vi "AixplorerMultiplexLoad.vi"() -> ()   [LabVIEW 2015]
uses:
  Tek shared libraries/ArbitraryFunctions/VImode.vi
  General Libraries/Sequences.lvlib
  Tek shared libraries/ArbitraryFunctions.lvlib
panel:
  in  "Stop Button":bool
  out "error out":errorcluster
  in  "resource name":refnum<k15>
  in  "?":enum32{"define waveforms", "load sequence"}(tab)
  in  "clear waveforms":bool
  out "Waveform Graph":dbl[][](graph)
  in  "define waveform":bool
  in  "Sequence Loop Initialization":T1(array[cluster])=[{"min"=0.0, "step"=0.25, "max"=1.0, "name"="Phase"}, {"min"=1.0, "step"=1.0, "max"=3.0, "name"="Harmonic"}]
  in  "Frequency LOW fundamental (Hz)":dbl=32467.5
  out "list waveform":string[][](table) caption="Loop variable"
  in  "N point":i32=960
  out "samplr rate":dbl
  in  "load sequence":bool
  in  "update voltage":bool
  in  "High Voltage (0.25)":dbl=0.5 format="%#_13g"
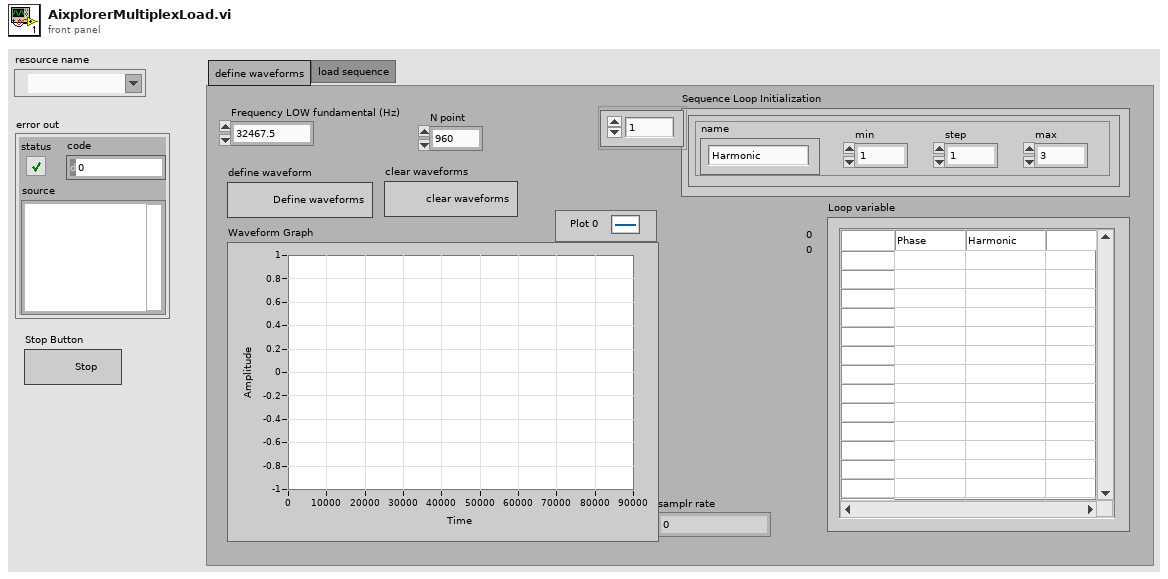
[diagram p1: front panel]
types:
  T1 = cluster{"min":dbl, "step":dbl, "max":dbl, "name":string}[]
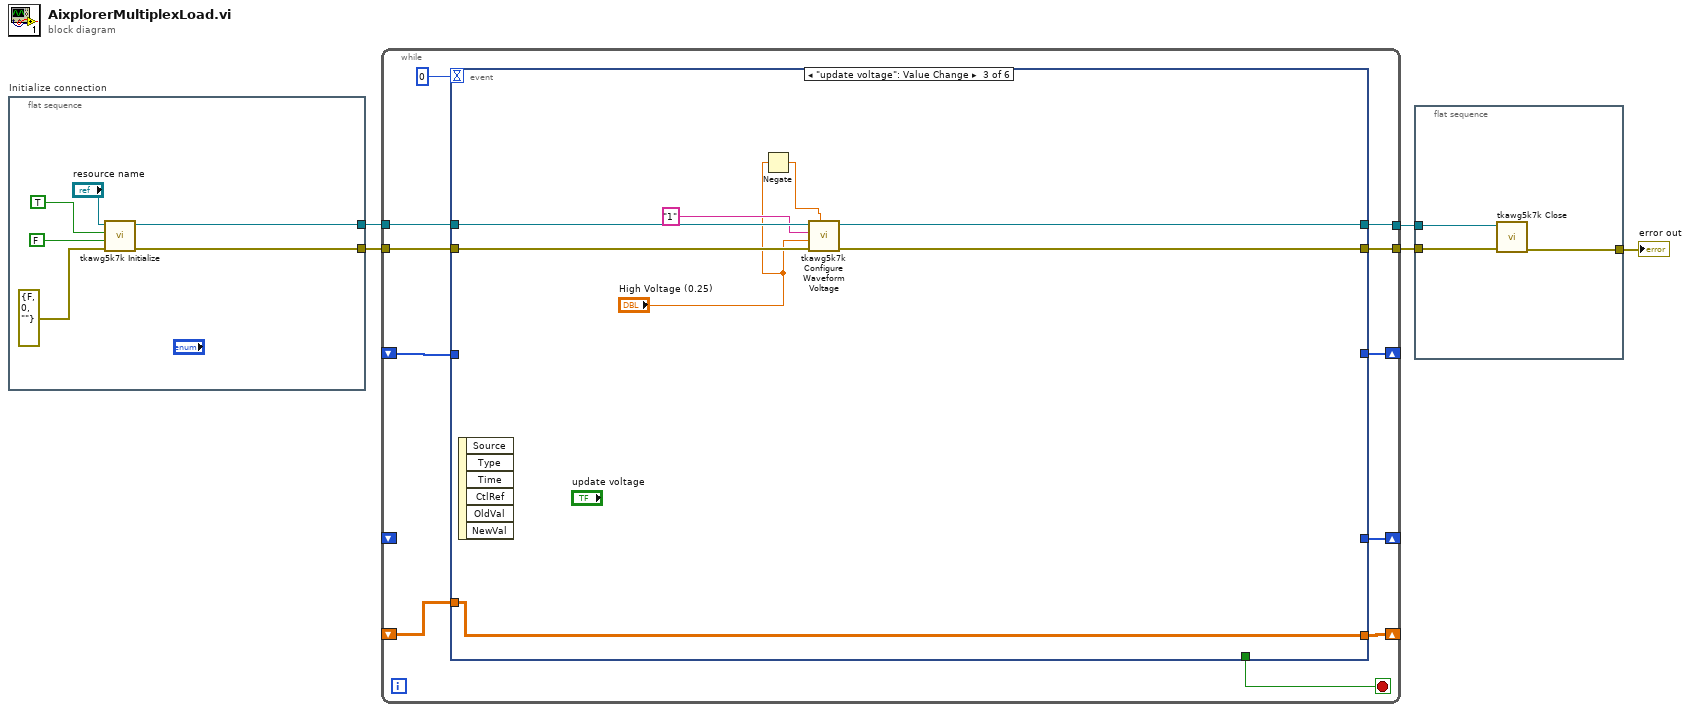
[diagram p0: block diagram]
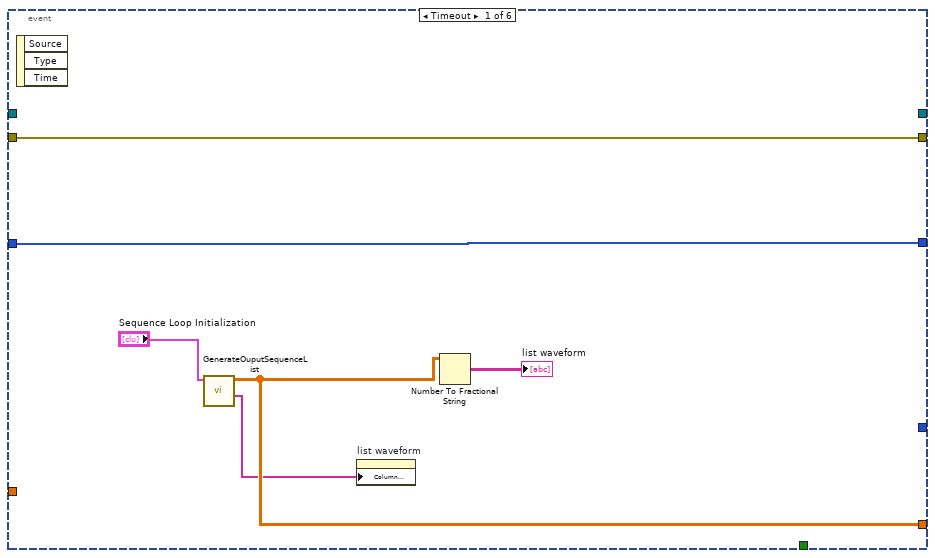
[diagram p2: hidden frame]
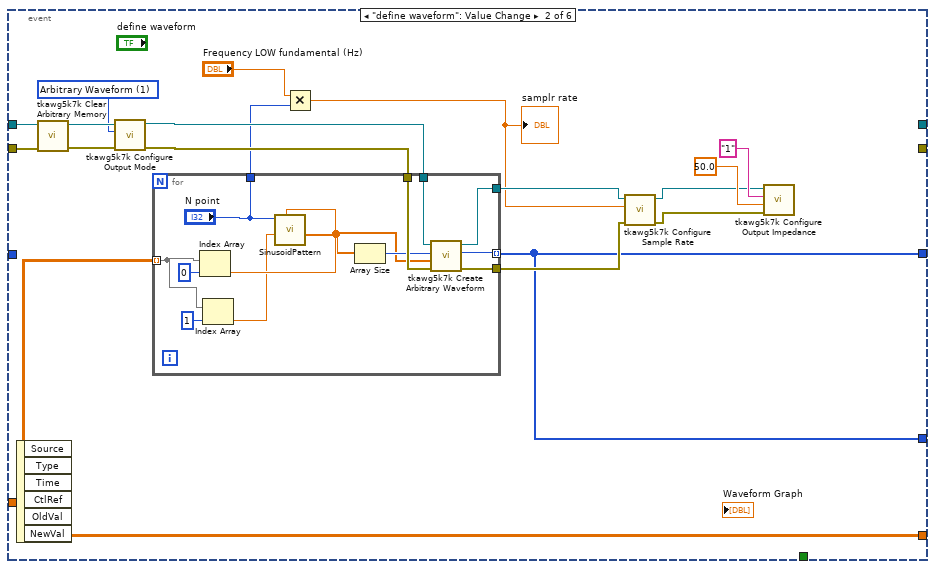
[diagram p3: hidden frame]
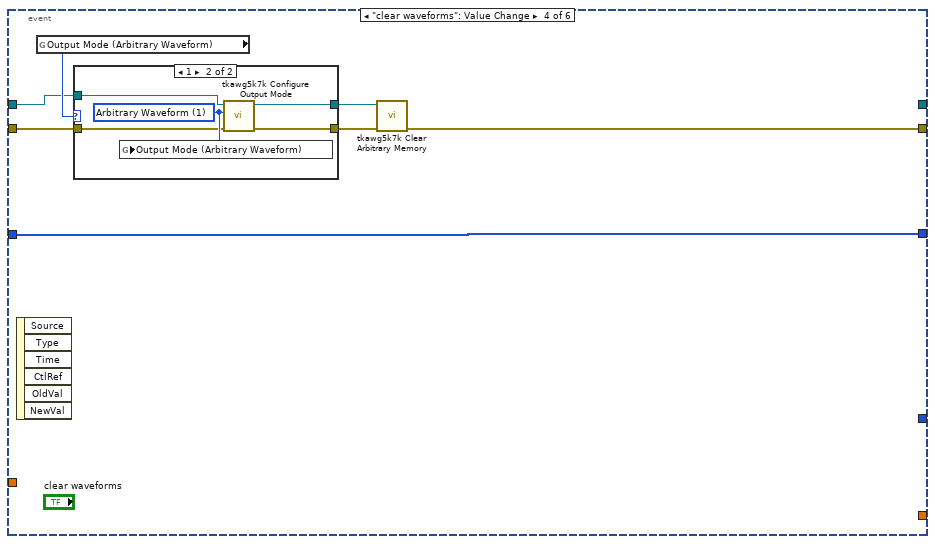
[diagram p4: hidden frame]
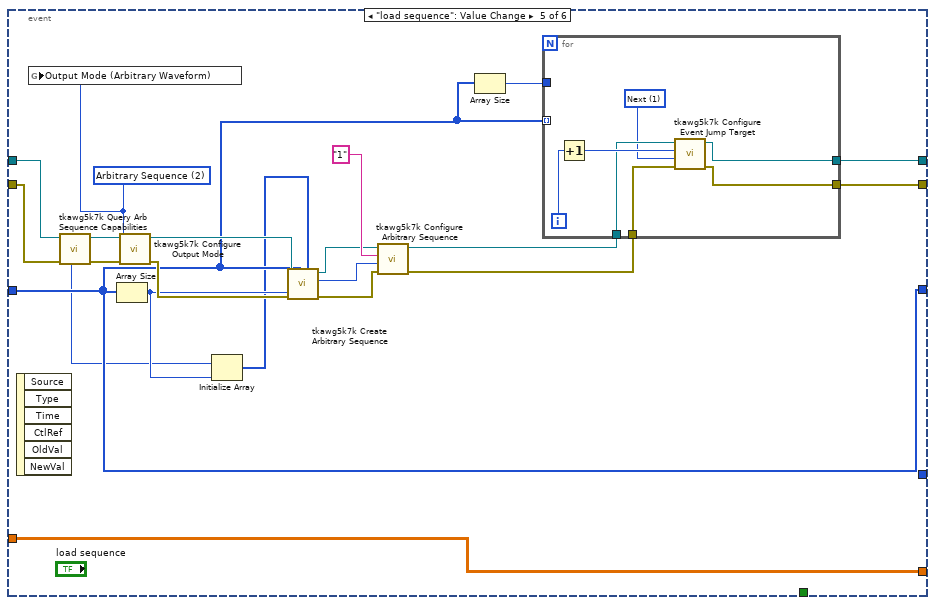
[diagram p6: hidden frame]
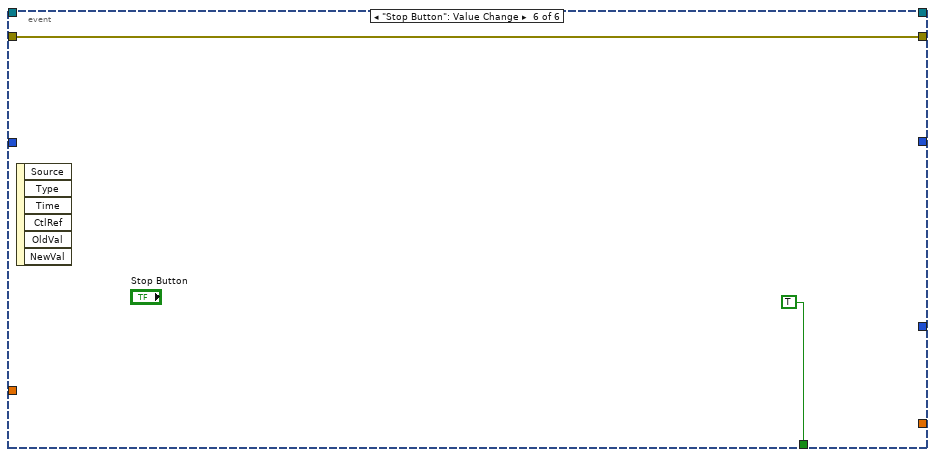
[diagram p7: hidden frame]
diagram:
  n1 = flat-sequence "Initialize connection" {
    tunnel: [w7] -> w5
    tunnel: [w6] -> w4
    frame #0 {
      n2 = call <instrlib>:"tkawg5k7k Initialize.vi"("error in (no error)"=errorcluster {"status"=FALSE, "code"=0, "source"=""}, "Reset Device (Yes)"=FALSE, "ID Query (Yes)"=TRUE, "resource name"="resource name") -> ("error out"=w6:errorcluster, "instrument handle out"=w7:refnum<k15>)  [unwired: 6 in]
    }
  }
  n3 = while {
    tunnel: w5 -> [w21]
    tunnel: w4 -> [w20]
    tunnel: [w22] -> w3
    tunnel: [w19] -> w2
    shift-right: [w16] -> _
    shift-left: _ -> [w15]
    shift-right: [w14] -> _
    shift-left: _ -> [w13]
    shift-right: [w12] -> _
    shift-left: _ -> [_]
    stop <- w17 stop-if-true
    n4 = event shown="[2] \"update voltage\": Value Change" {
      selector: _ -> [_ _ _ _ _ _]
      dyn-events: _ -> [_ _ _ _ _ _]
      timeout: 0 -> [_ _ _ _ _ _]
      tunnel: [_ _ w63 _ w91 _] -> w22
      tunnel: w21 -> [_ w45 w66 w73 w88 _]
      tunnel: w20 -> [w28 w44 w65 w72 w87 w110]
      tunnel: [w28 _ w62 w69 w94 w110] -> w19
      tunnel: [_ _ _ _ _ TRUE] -> w17
      tunnel: [w25 w46 w67 _ w102 _] -> w16
      tunnel: w15 -> [_ w46 w67 _ w102 _]
      tunnel: [w26 w32 _ w71 w93 _] -> w14
      tunnel: w13 -> [w26 _ _ w71 w93 _]
      tunnel: [_ w32 _ _ _ _] -> w12
      event Timeout {
        n5 = event-data() -> ()  [unwired: 1 in, 3 out]
        n6 = call "GenerateOuputSequenceList.vi"("input parameters"="Sequence Loop Initialization") -> ("output Names"=w23:string[], "output array"=w25:dbl[][])  [unwired: 9 in]
        n7 = property on="list waveform" class="Tbl (strict)"("Column Headers[]"=w23) -> ()  [unwired: 2 in, 2 out]
        n8 = Number To Fractional String(number=w25) -> (F-format string=→"list waveform":string[][])  [unwired: 3 in]
      }
      event "define waveform": Value Change {
        w39 = 1 items=["Arbitrary Waveform"=1, "Arbitrary Sequence"=2] ("Output Mode (Arbitrary Waveform)")
        n9 = event-data() -> ()  [unwired: 1 in, 6 out]
        n10 = call <instrlib>:"tkawg5k7k Clear Arbitrary Memory.vi"("error in (no error)"=w44, "instrument handle"=w45) -> ("error out"=w43:errorcluster, "instrument handle out"=w41:refnum<k15>)  [unwired: 8 in]
        n11 = call <instrlib>:"tkawg5k7k Configure Output Mode.vi"("error in (no error)"=w43, "Output Mode (Arbitrary Waveform)"=w39, "instrument handle"=w41) -> ("error out"=w42:errorcluster, "instrument handle out"=w40:refnum<k15>)  [unwired: 7 in]
        n12 = for {
          tunnel: w46 -> [w57] mode=indexing
          tunnel: w40 -> [w56]
          tunnel: w42 -> [w55]
          tunnel: [w53] -> w35
          tunnel: [w52] -> w36
          tunnel: [w51] -> w32 mode=indexing
          tunnel: ["N point"] -> w30
          n13 = Index Array(array=w57, index=0) -> (element=w50:dbl)
          n14 = Index Array(array=w57, index=1) -> (element=w49:dbl)
          n15 = call "SinusoidPattern.vi"("Phase (2pi unit)"=w50, "Nrep"=w49, "N point"="N point") -> ("Unit Pattern"=w48:dbl[])  [unwired: 7 in, 1 out]
          n16 = Array Size(array=w48) -> (size(s)=w54:i32)
          n17 = call <instrlib>:"tkawg5k7k Create Arbitrary Waveform.vi"("error in (no error)"=w55, "Waveform Data Array"=w48, "Waveform Size"=w54, "instrument handle"=w56) -> ("error out"=w53:errorcluster, "Waveform Handle"=w51:i32, "instrument handle out"=w52:refnum<k15>)  [unwired: 5 in]
        }
        n18 = Multiply(x="Frequency LOW fundamental (Hz)", y=w30) -> (x*y=w29:dbl)
        "samplr rate" <- w29
        n19 = call <instrlib>:"tkawg5k7k Configure Sample Rate.vi"("error in (no error)"=w35, "Sample Rate (5.0e+8)"=w29, "instrument handle"=w36) -> ("error out"=w34:errorcluster, "instrument handle out"=w33:refnum<k15>)  [unwired: 7 in]
        n20 = call <instrlib>:"tkawg5k7k Configure Output Impedance.vi"("error in (no error)"=w34, "Impedance (50.0)"=50.0, "Channel Name (\"1\")"="1" ("Channel Name (\"1\")"), "instrument handle"=w33) -> ()  [unwired: 6 in, 2 out]
      }
      event "update voltage": Value Change {
        n21 = event-data() -> ()  [unwired: 1 in, 6 out]
        n22 = Negate(x="High Voltage (0.25)") -> (-x=w60:dbl)
        n23 = call <instrlib>:"tkawg5k7k Configure Waveform Voltage.vi"("Low Voltage (-0.25)"=w60, "error in (no error)"=w65, "High Voltage (0.25)"="High Voltage (0.25)", "Channel Name (\"1\")"="1" ("Channel Name (\"1\")"), "instrument handle"=w66) -> ("error out"=w62:errorcluster, "instrument handle out"=w63:refnum<k15>)  [unwired: 5 in]
      }
      event "clear waveforms": Value Change {
        n24 = event-data() -> ()  [unwired: 1 in, 6 out]
        n25 = global read "VImode.vi" "Output Mode (Arbitrary Waveform)"() -> (w74:i32)
        n26 = case shown="1" w74 {
          tunnel: w73 -> [w76 w80]
          tunnel: w72 -> [w75 w79]
          tunnel: [w76 w78] -> w68
          tunnel: [w75 w77] -> w70
          frame 0, Default {
          }
          frame 1 {
            w81 = 1 items=["Arbitrary Waveform"=1, "Arbitrary Sequence"=2] ("Output Mode (Arbitrary Waveform)")
            n27 = global write "VImode.vi" "Output Mode (Arbitrary Waveform)"(w81) -> ()
            n28 = call <instrlib>:"tkawg5k7k Configure Output Mode.vi"("error in (no error)"=w79, "Output Mode (Arbitrary Waveform)"=w81, "instrument handle"=w80) -> ("error out"=w77:errorcluster, "instrument handle out"=w78:refnum<k15>)  [unwired: 7 in]
          }
        }
        n29 = call <instrlib>:"tkawg5k7k Clear Arbitrary Memory.vi"("error in (no error)"=w70, "instrument handle"=w68) -> ("error out"=w69:errorcluster)  [unwired: 8 in, 1 out]
      }
      event "load sequence": Value Change {
        w97 = 2 items=["Arbitrary Waveform"=1, "Arbitrary Sequence"=2] ("Output Mode (Arbitrary Waveform)")
        n30 = event-data() -> ()  [unwired: 1 in, 6 out]
        n31 = global write "VImode.vi" "Output Mode (Arbitrary Waveform)"(w97) -> ()
        n32 = call <instrlib>:"tkawg5k7k Query Arb Sequence Capabilities.vi"("error in (no error)"=w87, "instrument handle"=w88) -> ("error out"=w86:errorcluster, "instrument handle out"=w85:refnum<k15>, "Max Loop Count"=w83:i32)  [unwired: 4 in, 3 out]
        n33 = Array Size(array=w93) -> (size(s)=w84:i32)
        n34 = call <instrlib>:"tkawg5k7k Configure Output Mode.vi"("error in (no error)"=w86, "Output Mode (Arbitrary Waveform)"=w97, "instrument handle"=w85) -> ("error out"=w98:errorcluster, "instrument handle out"=w99:refnum<k15>)  [unwired: 7 in]
        n35 = Initialize Array(w83, w84) -> (w82:i32[])
        n36 = call <instrlib>:"tkawg5k7k Create Arbitrary Sequence.vi"("Loop Counts Array"=w82, "Waveform Handles Array"=w93, "error in (no error)"=w98, "Sequence Length"=w84, "instrument handle"=w99) -> ("error out"=w89:errorcluster, "Sequence Handle"=w101:i32, "instrument handle out"=w90:refnum<k15>)  [unwired: 4 in]
        n37 = call <instrlib>:"tkawg5k7k Configure Arbitrary Sequence.vi"("error in (no error)"=w89, "Sequence Handle"=w101, "Channel Name (\"1\")"="1" ("Channel Name (\"1\")"), "instrument handle"=w90) -> ("error out"=w95:errorcluster, "instrument handle out"=w92:refnum<k15>)  [unwired: 6 in]
        n38 = Array Size(array=w93) -> (size(s)=w96:i32)
        n39 = for {
          tunnel: w93 -> [_] mode=indexing
          tunnel: w96 -> [_]
          tunnel: w95 -> [w107]
          tunnel: [w106] -> w94
          tunnel: w92 -> [w105]
          tunnel: [w104] -> w91
          i -> [w109]
          w103 = 1 items=["Index", "Next", "Off"] ("Jump Type (Off)")
          n40 = Increment(x=w109) -> (x+1=w108:i32)
          n41 = call <instrlib>:"tkawg5k7k Configure Event Jump Target.vi"("error in (no error)"=w107, "Jump Type (Off)"=w103, "Element (1)"=w108, "instrument handle"=w105) -> ("error out"=w106:errorcluster, "instrument handle out"=w104:refnum<k15>)  [unwired: 6 in]
        }
      }
      event "Stop Button": Value Change {
        n42 = event-data() -> ()  [unwired: 1 in, 6 out]
      }
    }
  }
  n43 = flat-sequence {
    tunnel: w3 -> [w112]
    tunnel: w2 -> [w114]
    tunnel: [w113] -> w1
    frame #0 {
      n44 = call <instrlib>:"tkawg5k7k Close.vi"("error in (no error)"=w114, "instrument handle"=w112) -> ("error out"=w113:errorcluster)  [unwired: 9 in]
    }
  }
  "error out" <- w1
